vi "UI Page Disply_Error Occur.vi"(8 "error in (no error)":errorcluster, 10 "Tab Main":refnum<vi>, 11 "MPC_AutoInspection in":refnum<class "MPC_AutoInspection.lvclass">) -> (0 "error out":errorcluster, 3 "MPC_AutoInspection out":refnum<class "MPC_AutoInspection.lvclass">)   [LabVIEW 2019, in "MPC_AutoInspection.lvclass"]
uses:
  MPC_AutoInspection.lvclass
  Main Class.lvclass
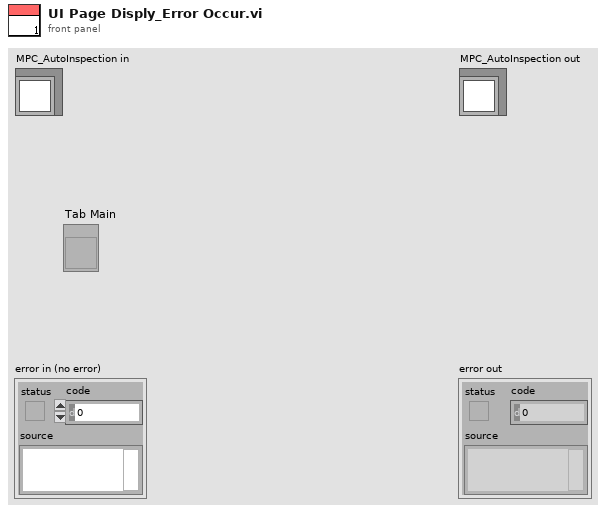
[diagram p1: front panel]
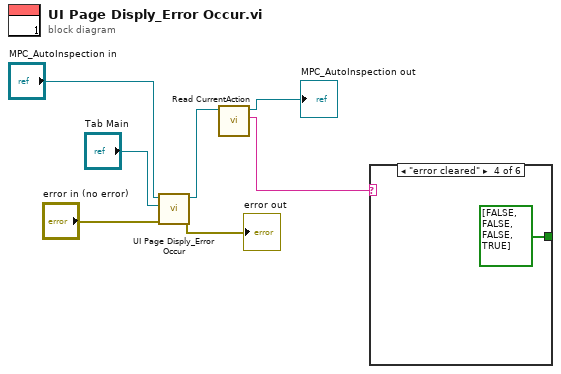
[diagram p0: block diagram]
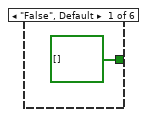
[diagram p2: hidden frame]
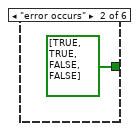
[diagram p3: hidden frame]
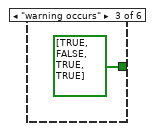
[diagram p4: hidden frame]
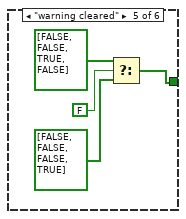
[diagram p5: hidden frame]
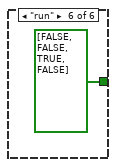
[diagram p6: hidden frame]
diagram:
  n1 = call-parent "UI Page Disply_Error Occur.vi"("error in (no error)"="error in (no error)", "Tab Main"="Tab Main", "Main Class in"="MPC_AutoInspection in") -> ("error out"=→"error out":errorcluster, "Main Class out"=w3:refnum<class "MPC_AutoInspection.lvclass">)  [unwired: 7 in]
  n2 = call-dynamic "Read CurrentAction.vi"("Main Process Class in"=w3) -> ("CurrentAction"=w1:string, "Main Process Class out"=→"MPC_AutoInspection out":refnum<class "MPC_AutoInspection.lvclass">)  [unwired: 8 in, 1 out]
  n3 = case shown="\"error cleared\"" w1 {
    tunnel: [bool[] [] bool[] [TRUE, TRUE, FALSE, FALSE] bool[] [TRUE, FALSE, TRUE, TRUE] bool[] [FALSE, FALSE, FALSE, TRUE] w14 bool[] [FALSE, FALSE, TRUE, FALSE]] -> _
    frame "False", Default {
    }
    frame "error occurs" {
    }
    frame "warning occurs" {
    }
    frame "error cleared" {
    }
    frame "warning cleared" {
      n4 = Select(t=bool[] [FALSE, FALSE, TRUE, FALSE], s=FALSE, f=bool[] [FALSE, FALSE, FALSE, TRUE]) -> (s? t:f=w14:bool[])
    }
    frame "run" {
    }
  }
